vi "Draw Horizon.vi"(7 "attitude (rad)":T1, 9 "draw options":T2={"Text Color"=16777238, "Wing Color"=16751616, "Dial Outline Color"=13816530, "Sky Color"=3381759, "Ground Color"=8213043, "Horizon Line Color"=16777225, "Outline Color"=0, "Dial Background Color"=5987163, "Draw Wings"=TRUE, "Draw Text"=TRUE, "Font Name"="Helvetica", "Angle units"=enum."Radians"}, 10 "draw area state":T4, 11 "picture in":picture) -> (3 "picture out":picture)   [LabVIEW 2017, in "NI_Robotics_Attitude Picture.lvlib"]
uses:
  <vilib>/robotics/Controls/Attitude Indicator/Attitude Picture/NI_Robotics_Attitude Picture.lvlib
  <vilib>/robotics/Controls/Attitude Indicator/Attitude Picture/Draw Area State.ctl
  <vilib>/Utility/miscctls.llb/LVBoundsTypeDef.ctl
  <vilib>/robotics/Controls/Attitude Indicator/Attitude Picture/Draw Options.ctl
  <vilib>/robotics/Controls/Utilities/Angle Units.ctl
  <vilib>/robotics/Controls/Attitude Indicator/Attitude Picture/Attitude.ctl
  <vilib>/Analysis/coordinate.llb/2D Cartesian Coordinate Rotation (Array).vi
  <vilib>/Utility/AngleManip/Degrees to Radians (Array DBL).vi
  <vilib>/Utility/AngleManip/Degrees to Radians (Scalar DBL).vi
  <vilib>/Analysis/NI_AALPro.lvlib
  <vilib>/Utility/AngleManip/NI_AngleManipulation.lvlib
  <vilib>/robotics/Controls/Utilities/NI_Robotics_Control Utilities.lvlib
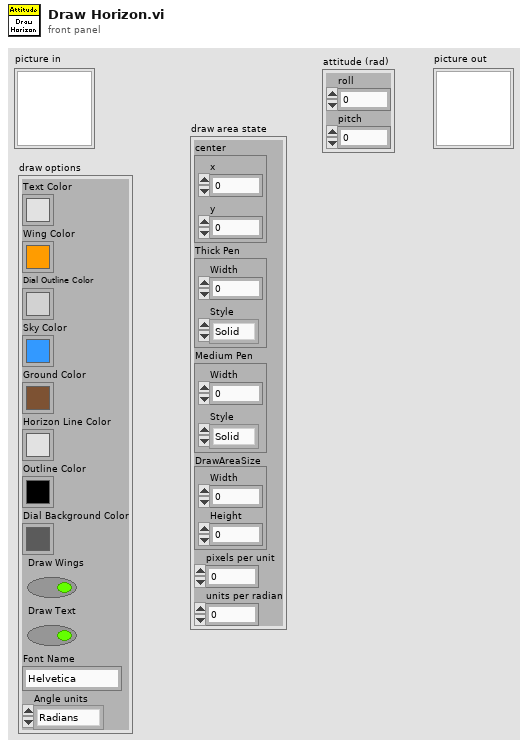
[diagram p1: front panel]
types:
  T1 = typedef "NI_Robotics_Attitude Picture.lvlib/Attitude.ctl" = cluster{"roll":dbl, "pitch":dbl}
  T2 = typedef "NI_Robotics_Attitude Picture.lvlib/Draw Options.ctl" = cluster{"Text Color":u32, "Wing Color":u32, "Dial Outline Color":u32, "Sky Color":u32, "Ground Color":u32, "Horizon Line Color":u32, "Outline Color":u32, "Dial Background Color":u32, "Draw Wings":bool, "Draw Text":bool, "Font Name":string, "Angle units":T3}
  T3 = typedef "NI_Robotics_Control Utilities.lvlib/Angle Units.ctl" = enum16{"Radians", "Degrees"}
  T4 = typedef "NI_Robotics_Attitude Picture.lvlib/Draw Area State.ctl" = cluster{"center":cluster{"x":i16, "y":i16}, "Thick Pen":cluster{"Width":u16, "Style":enum32{"Solid", "Dash", "Dot", "DashDot", "DashDotDot"}}, "Medium Pen":cluster{"Width":u16, "Style":enum32{"Solid", "Dash", "Dot", "DashDot", "DashDotDot"}}, "DrawAreaSize":T5, "pixels per unit":dbl, "units per radian":dbl}
  T5 = typedef "LVBoundsTypeDef.ctl" = cluster{"Width":u32, "Height":u32}
  T6 = cluster{"Width":u16, "Style":enum32{"Solid", "Dash", "Dot", "DashDot", "DashDotDot"}}
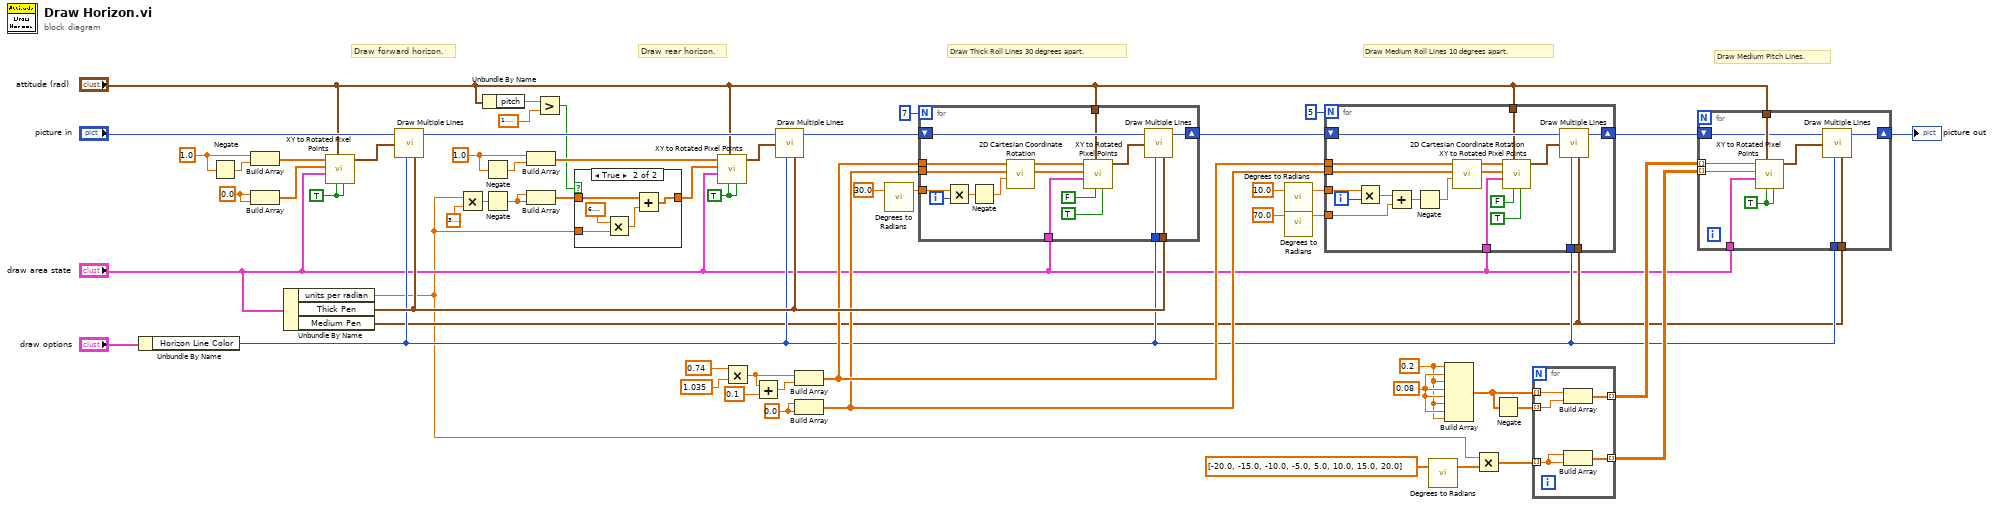
[diagram p0: block diagram]
diagram:
  w19 = 0.08
  w18 = 0.2
  w38 = 0.0 ("element")
  w41 = TRUE ("use pitch")
  w42 = TRUE ("use pitch")
  w49 = 1.0 ("element")
  w56 = 0.0 ("element")
  w57 = 1.0 ("element")
  # "Draw Medium Pitch Lines."
  # "Draw Medium Roll Lines 10 degrees apart."
  # "Draw Thick Roll Lines 30 degrees apart."
  # "Draw rear horizon."
  # "Draw forward horizon."
  n1 = Unbundle By Name("draw options") -> ("Horizon Line Color"=w11:u32)
  n2 = Negate(x=w57) -> (-x=w58:dbl)
  n3 = Build Array(w57, w58) -> (w53:dbl[])
  n4 = Build Array(w56, w56) -> (w52:dbl[])
  n5 = Unbundle By Name("draw area state") -> ("units per radian"=w1:dbl, "Thick Pen"=w39:T6, "Medium Pen"=w10:T6)
  n6 = call <vilib>:"XY to Rotated Pixel Points.vi"("use roll"=w42, "use pitch"=w42, "attitude (rad)"="attitude (rad)", "draw area state"="draw area state", "unrotated y (units)"=w52, "unrotated x (units)"=w53) -> ("rotated pixel points"=w51:cluster{"x":i16, "y":i16}[])  [unwired: 5 in]
  n7 = call <vilib>:"Draw Multiple Lines.vi"("picture"="picture in", "line endpoints"=w51, "color(black)"=w11, "pen"=w39) -> ("new picture"=w44:picture)  [unwired: 5 in]
  n8 = Multiply(x=w1, y=3.141592653589793) -> (x*y=w47:dbl)
  n9 = Unbundle By Name("attitude (rad)") -> ("pitch"=w5:dbl)
  n10 = Negate(x=w49) -> (-x=w48:dbl)
  n11 = Negate(x=w47) -> (-x=w45:dbl)
  n12 = Build Array(w49, w48) -> (w50:dbl[])
  n13 = Build Array(w45, w45) -> (w4:dbl[])
  n14 = Greater?(x=w5, y=1.5707963267948966) -> (0:w2:bool)
  n15 = case shown="True" w2 {
    tunnel: w4 -> [w59 w64]
    tunnel: [w59 w63] -> w3
    tunnel: w1 -> [_ w61]
    frame False {
    }
    frame True {
      n16 = Multiply(x=6.283185307179586, y=w61) -> (x*y=w60:dbl)
      n17 = Add(x=w64, y=w60) -> (x+y=w63:dbl[])
    }
  }
  n18 = call <vilib>:"XY to Rotated Pixel Points.vi"("use roll"=w41, "use pitch"=w41, "attitude (rad)"="attitude (rad)", "draw area state"="draw area state", "unrotated y (units)"=w3, "unrotated x (units)"=w50) -> ("rotated pixel points"=w43:cluster{"x":i16, "y":i16}[])  [unwired: 5 in]
  n19 = Multiply(x=0.74, y=1.035) -> (x*y=w35:dbl)
  n20 = Add(x=w35, y=0.1) -> (x+y=w33:dbl)
  n21 = call <vilib>:"Draw Multiple Lines.vi"("picture"=w44, "line endpoints"=w43, "color(black)"=w11, "pen"=w39) -> ("new picture"=w40:picture)  [unwired: 5 in]
  n22 = Build Array(w35, w33) -> (w23:dbl[])
  n23 = Build Array(w38, w38) -> (w22:dbl[])
  n24 = call-poly <vilib>:"Degrees to Radians.vi"("angle (deg)"=30.0) -> ("angle (rad)"=w31:dbl)  [unwired: 2 in]
  n25 = for {
    N: 7 -> [_]
    shift-right: [w80] -> w29
    shift-left: w40 -> [w81]
    tunnel: "draw area state" -> [w79]
    tunnel: "attitude (rad)" -> [w78]
    tunnel: w11 -> [w65]
    tunnel: w39 -> [w74]
    tunnel: w23 -> [w71]
    tunnel: w22 -> [w70]
    tunnel: w31 -> [w73]
    i -> [w72]
    n26 = Multiply(x=w73, y=w72) -> (x*y=w69:dbl)
    n27 = Negate(x=w69) -> (-x=w66:dbl)
    n28 = call-poly <vilib>:"2D Cartesian Coordinate Rotation.vi"("theta"=w66, "Y"=w70, "X"=w71) -> ("Y Out"=w67:dbl[], "X Out"=w68:dbl[])  [unwired: 6 in, 1 out]
    n29 = call <vilib>:"XY to Rotated Pixel Points.vi"("use roll"=TRUE, "use pitch"=FALSE, "attitude (rad)"=w78, "draw area state"=w79, "unrotated y (units)"=w67, "unrotated x (units)"=w68) -> ("rotated pixel points"=w77:cluster{"x":i16, "y":i16}[])  [unwired: 5 in]
    n30 = call <vilib>:"Draw Multiple Lines.vi"("picture"=w81, "line endpoints"=w77, "color(black)"=w65, "pen"=w74) -> ("new picture"=w80:picture)  [unwired: 5 in]
  }
  n31 = call-poly <vilib>:"Degrees to Radians.vi"("angle (deg)"=10.0) -> ("angle (rad)"=w26:dbl)  [unwired: 2 in]
  n32 = call-poly <vilib>:"Degrees to Radians.vi"("angle (deg)"=70.0) -> ("angle (rad)"=w24:dbl)  [unwired: 2 in]
  n33 = for {
    N: 5 -> [_]
    shift-right: [w99] -> w17
    shift-left: w29 -> [w100]
    tunnel: w26 -> [w98]
    tunnel: w24 -> [w95]
    tunnel: "draw area state" -> [w90]
    tunnel: w11 -> [w86]
    tunnel: w10 -> [w85]
    tunnel: w23 -> [w84]
    tunnel: w22 -> [w83]
    tunnel: "attitude (rad)" -> [w82]
    i -> [w97]
    n34 = Multiply(x=w98, y=w97) -> (x*y=w96:dbl)
    n35 = Add(x=w96, y=w95) -> (x+y=w94:dbl)
    n36 = Negate(x=w94) -> (-x=w93:dbl)
    n37 = call-poly <vilib>:"2D Cartesian Coordinate Rotation.vi"("theta"=w93, "Y"=w83, "X"=w84) -> ("Y Out"=w91:dbl[], "X Out"=w92:dbl[])  [unwired: 6 in, 1 out]
    n38 = call <vilib>:"XY to Rotated Pixel Points.vi"("use roll"=TRUE, "use pitch"=FALSE, "attitude (rad)"=w82, "draw area state"=w90, "unrotated y (units)"=w91, "unrotated x (units)"=w92) -> ("rotated pixel points"=w87:cluster{"x":i16, "y":i16}[])  [unwired: 5 in]
    n39 = call <vilib>:"Draw Multiple Lines.vi"("picture"=w100, "line endpoints"=w87, "color(black)"=w86, "pen"=w85) -> ("new picture"=w99:picture)  [unwired: 5 in]
  }
  n40 = call-poly <vilib>:"Degrees to Radians.vi"("angles (deg)"=dbl[] [-20.0, -15.0, -10.0, -5.0, 5.0, 10.0, 15.0, 20.0]) -> ("angles (rad)"=w20:dbl[])  [unwired: 2 in]
  n41 = Build Array(w18, w19, w18, w19, w19, w18, w19, w18) -> (w16:dbl[])
  n42 = Multiply(x=w1, y=w20) -> (x*y=w14:dbl[])
  n43 = Negate(x=w16) -> (-x=w15:dbl[])
  n44 = for {
    tunnel: w16 -> [w105] mode=indexing
    tunnel: w15 -> [w104] mode=indexing
    tunnel: w14 -> [w103] mode=indexing
    tunnel: [w102] -> w13 mode=indexing
    tunnel: [w101] -> w12 mode=indexing
    n45 = Build Array(w105, w104) -> (w102:dbl[])
    n46 = Build Array(w103, w103) -> (w101:dbl[])
  }
  n47 = for {
    tunnel: w13 -> [w115] mode=indexing
    tunnel: w12 -> [w114] mode=indexing
    tunnel: "draw area state" -> [w113]
    tunnel: "attitude (rad)" -> [w112]
    tunnel: w11 -> [w109]
    tunnel: w10 -> [w108]
    shift-right: [w107] -> w9
    shift-left: w17 -> [w111]
    w106 = TRUE ("use pitch")
    n48 = call <vilib>:"XY to Rotated Pixel Points.vi"("use roll"=w106, "use pitch"=w106, "attitude (rad)"=w112, "draw area state"=w113, "unrotated y (units)"=w114, "unrotated x (units)"=w115) -> ("rotated pixel points"=w110:cluster{"x":i16, "y":i16}[])  [unwired: 5 in]
    n49 = call <vilib>:"Draw Multiple Lines.vi"("picture"=w111, "line endpoints"=w110, "color(black)"=w109, "pen"=w108) -> ("new picture"=w107:picture)  [unwired: 5 in]
  }
  "picture out" <- w9
